vi "Read PUBCOMP.vi"(8 "error in (no error)":errorcluster, 11 "connection ID":refnum<k5>) -> (0 "error out":errorcluster, 2 "Message ID":u16=10 format="%x", 3 "connection ID out":refnum<k5>)   [LabVIEW 2020, in "DAQIO MQTT.lvlib"]
doc: "© 2015 - daq.io, LLC - Peter Adelhardt"
uses:
  DAQIO MQTT.lvlib
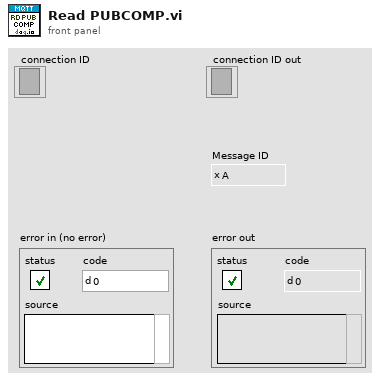
[diagram p1: front panel]
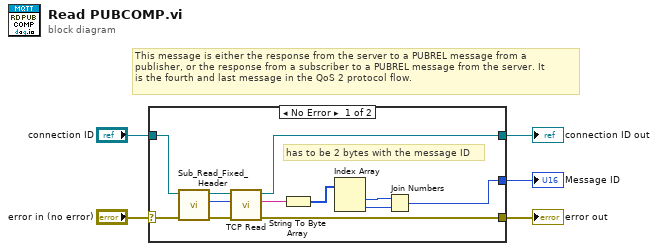
[diagram p0: block diagram]
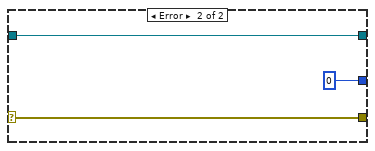
[diagram p2: hidden frame]
diagram:
  # "This message is either the response from the server to a PUBREL message from a\npublisher, or the response from a subscriber to a PUBREL message from the server. It\nis the fourth and last message in the QoS 2 protocol flow."
  n1 = case shown="No Error" "error in (no error)" {
    selector: "error in (no error)" -> [w13 w20]
    tunnel: [w12 w20] -> w4
    tunnel: "connection ID" -> [w8 w19]
    tunnel: [w7 u16 0] -> w2
    tunnel: [w6 w19] -> w1
    frame No Error {
      # "has to be 2 bytes with the message ID"
      n2 = call "Sub_Read_Fixed_Header.vi"("error in (no error)"=w13, "connection ID"=w8) -> ("error out"=w9:errorcluster, "Remaining Length"=w11:u32, "connection ID out"=w10:refnum<k5>)  [unwired: 3 in, 4 out]
      n3 = call "TCP Read.vi"("error in (no error)"=w9, "bytes to read"=w11, "connection ID"=w10) -> ("error out"=w12:errorcluster, "data out"=w17:string, "connection ID out"=w6:refnum<k5>)  [unwired: 6 in]
      n4 = String To Byte Array(string=w17) -> (unsigned byte array=w16:u8[])
      n5 = Index Array(array=w16) -> (element #1=w14:u8, element #2=w15:u8)  [unwired: 2 in]
      n6 = Join Numbers(hi=w14, lo=w15) -> ((hi.lo)=w7:u16)
    }
    frame Error {
    }
  }
  "error out" <- w4
  "connection ID out" <- w1
  "Message ID" <- w2
